vi "S8300E_WriteSN.vi"() -> ()   [LabVIEW 2011]
panel:
  out "log1":string
  out "Debug View":string
  out "UUT SN":string
  out "CMD-LIST":cluster{string, string, string, string}[](array[cluster])
  out "log msg":string
  out "VISA resource name out":refnum<visa-resource-name>
  out "BEGIN TIME":u32
  out "進行狀況":string
  # "2014-12-15"
  # "S8300E Program SN (接UART COM9)"
  # "Error Code:SN-SET"
  # "Set Serial Number to BIOS Flash"
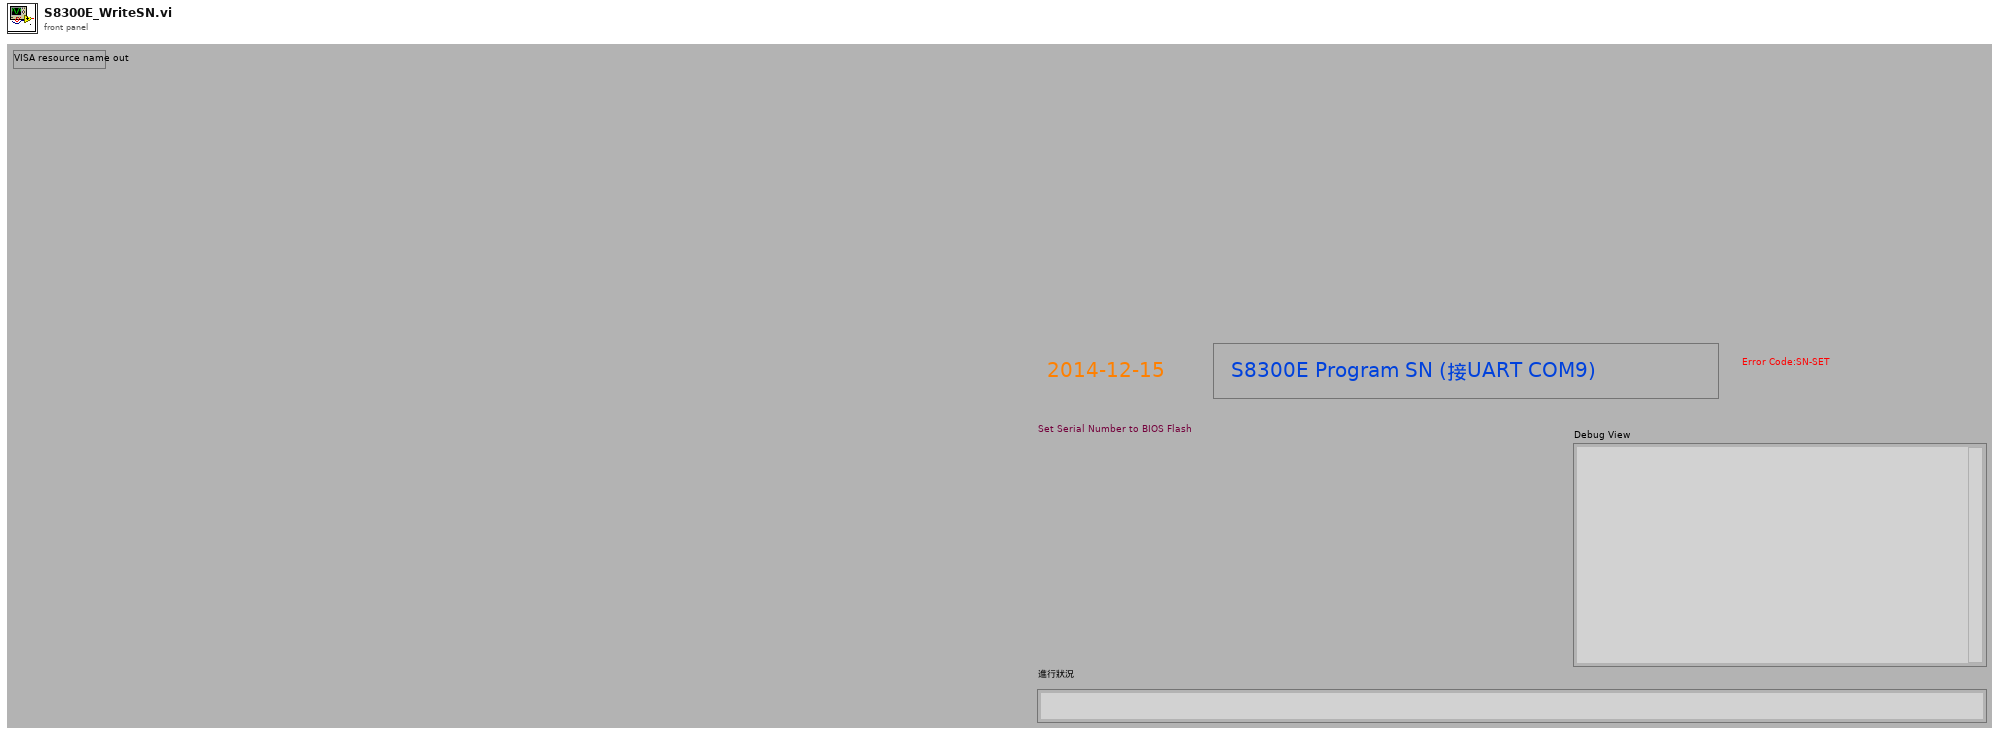
[diagram p1: front panel]
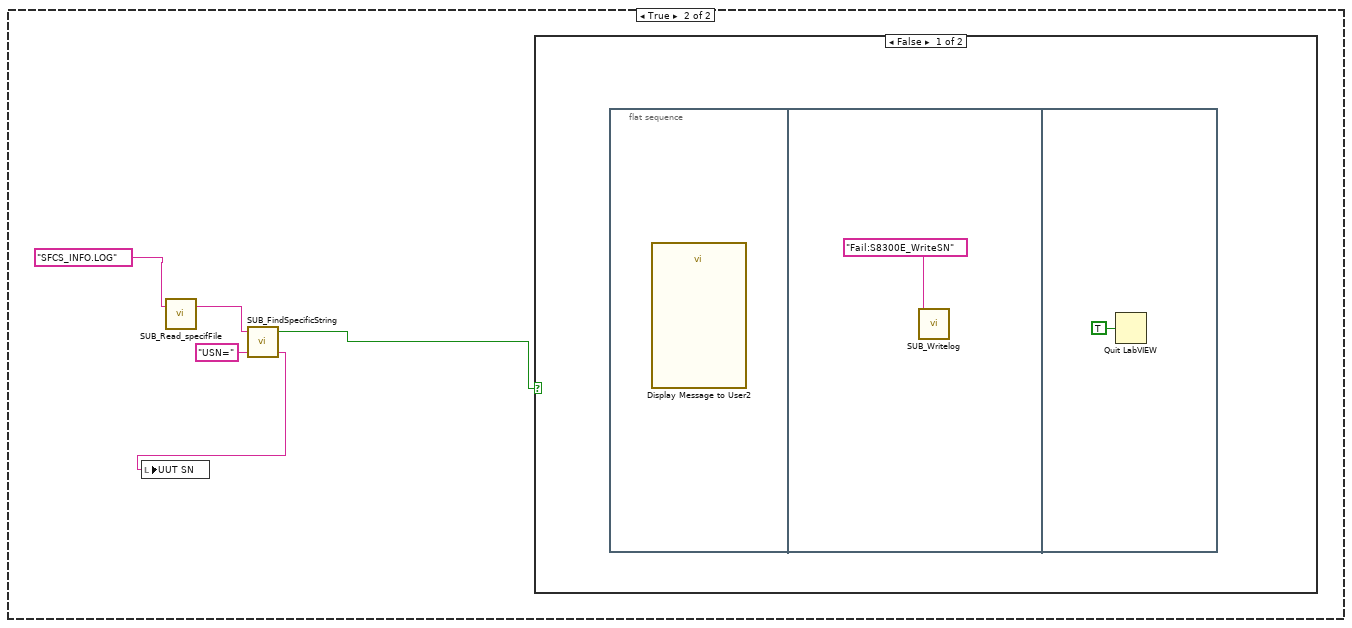
[diagram p3: hidden frame]
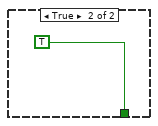
[diagram p7: hidden frame]
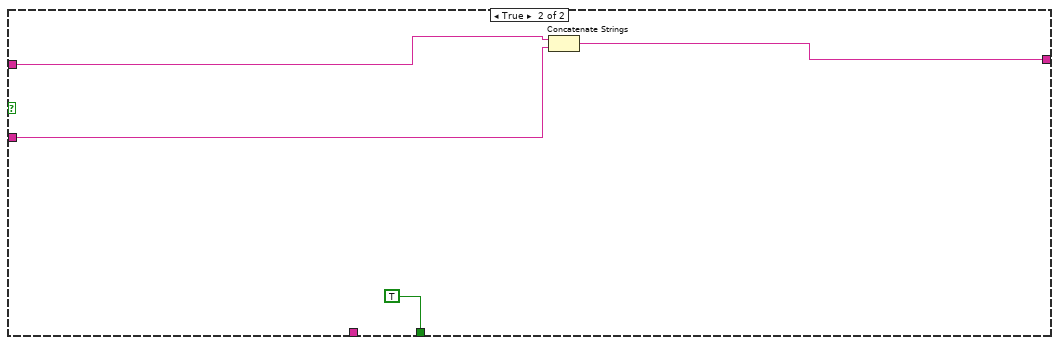
[diagram p9: hidden frame]
diagram:
  n1 = flat-sequence {
    frame #0 {
      n2 = Tick Count (ms)() -> (millisecond timer value=→"BEGIN TIME":u32)
    }
    frame #1 {
      w2 = ""
      n3 = property on="進行狀況" class="Str"("Blinking"=TRUE) -> ()  [unwired: 2 in, 2 out]
      "進行狀況" <- "進入測試準備中...." ("進行狀況")
      "UUT SN" <- w2
      "Debug View" <- w2
    }
    frame #2 {
      n4 = call "SUB_SearchFile_inFolder.vi"("Search Filename in Folder"="S8300E_sfcs_misc.txt") -> ("File Existing True/Flase"=w5:bool)  [unwired: 1 in]
      n5 = case shown="False" w5 {
        frame False {
          n6 = flat-sequence {
            frame #0 {
              n7 = call "Display Message to User"() -> ()  [unwired: 10 in, 2 out]
            }
            frame #1 {
              n8 = call "SUB_Writelog.vi"("Pass/Fail"="Fail:S8300E_WriteSN") -> ()  [unwired: 2 in]
            }
            frame #2 {
              n9 = Quit LabVIEW(quit? (T)=TRUE) -> ()
            }
          }
        }
        frame True {
        }
      }
    }
    frame #3 {
    }
    frame #4 {
      n10 = call "SUB_SearchFile_inFolder.vi"("Search Filename in Folder"="SFCS_INFO.LOG") -> ("File Existing True/Flase"=w9:bool)  [unwired: 1 in]
      n11 = case shown="False" w9 {
        frame False {
          n12 = flat-sequence {
            frame #0 {
              n13 = call "Display Message to User3"() -> ()  [unwired: 10 in, 2 out]
            }
            frame #1 {
              n14 = call "SUB_Writelog.vi"("Pass/Fail"="Fail:S8300E_WriteSN") -> ()  [unwired: 2 in]
            }
            frame #2 {
              n15 = Quit LabVIEW(quit? (T)=TRUE) -> ()
            }
          }
        }
        frame True {
          n16 = call "SUB_Read_specifFile.vi"("name or relative path"="SFCS_INFO.LOG" ("Search Filename in Folder")) -> ("text"=w16:string)  [unwired: 1 in, 1 out]
          n17 = call "SUB_FindSpecificString.vi"("Find this String"="USN=", "String data"=w16) -> ("before \"; \" string"=w14:string, "Found"=w13:bool)  [unwired: 2 in]
          n18 = local write "UUT SN"(w14) -> ()
          n19 = case shown="False" w13 {
            frame False {
              n20 = flat-sequence {
                frame #0 {
                  n21 = call "Display Message to User2"() -> ()  [unwired: 10 in, 2 out]
                }
                frame #1 {
                  n22 = call "SUB_Writelog.vi"("Pass/Fail"="Fail:S8300E_WriteSN") -> ()  [unwired: 2 in]
                }
                frame #2 {
                  n23 = Quit LabVIEW(quit? (T)=TRUE) -> ()
                }
              }
            }
            frame True {
            }
          }
        }
      }
    }
    frame #5 {
      n24 = local read "UUT SN"() -> (w23:string)
      n25 = Concatenate Strings("PASSED=", w23) -> (w22:string)
      n26 = Concatenate Strings("PASSED=", w23) -> (w25:string)
      n27 = Concatenate Strings("./ser.sh -w -f  ", w23, "\r") -> (w41:string)
      n28 = Concatenate Strings("./ser.sh -r -f  ", "\r") -> (w38:string)
      n29 = Concatenate Strings("./ser.sh -r -d ", "\r") -> (w35:string)
      n30 = Bundle(w41, "PASSED=", "Set Serial Number to BIOS Flash", "SN-SET") -> (w30:cluster{string, string, string, string})  [unwired: 1 in]
      n31 = Bundle(w38, w25, "Get Serial Number from BIOS Flash", "SN-BIOS") -> ()  [unwired: 1 in, 1 out]
      n32 = Bundle(w35, w22, "Get Serial Number from DMI table", "SN-DMI") -> ()  [unwired: 1 in, 1 out]
      n33 = Build Array(w30) -> (→"CMD-LIST":cluster{string, string, string, string}[])
    }
    frame #6 {
      n34 = call "SUB_COM1_CLOSE.vi"("VISA resource name"=refnum<visa-resource-name> "COM9") -> ()  [unwired: 3 in]
    }
    frame #7 {
      n35 = call "SUB_COM9_INIT.vi"("baud rate"=u32 115200) -> ("VISA resource name out"=w47:refnum<visa-resource-name>)  [unwired: 1 in, 1 out]
      "VISA resource name out" <- w47
      n36 = call "SUB_COM1Wrt.vi"("VISA resource name"=w47, "write buffer"="\r") -> ("duplicate VISA resource name"=w44:refnum<visa-resource-name>)  [unwired: 1 in, 1 out]
      n37 = call "SUB_ContinueCom1Read.vi"("Numeric"=1200, "duplicate VISA resource name 2"=w44) -> ()  [unwired: 1 in, 3 out]
    }
    frame #8 {
      n38 = case shown="True" TRUE {
        frame False {
        }
        frame True {
          n39 = while {
            stop <- w57 stop-if-true
            n40 = local read "VISA resource name out"() -> (w51:refnum<visa-resource-name>)
            n41 = call "SUB_COM1Wrt.vi"("VISA resource name"=w51, "write buffer"="\r") -> ("duplicate VISA resource name"=w56:refnum<visa-resource-name>)  [unwired: 1 in, 1 out]
            n42 = Tick Count (ms)() -> (millisecond timer value=w55:u32)
            n43 = call "SUB_READ_COM1_FindString_timeout.vi"("Find this String"="s8300e_func_test", "Timeout Seccond"=1.0, "Begin time"=w55, "duplicate VISA resource name 2"=w56) -> ("Output String"=w50:string, "Found String"=w52:bool)  [unwired: 1 in, 1 out]
            "log1" <- w50
            n44 = local write "Debug View"(w50) -> ()
            n45 = case shown="False" w52 {
              tunnel: [w60 TRUE] -> w57
              tunnel: w50 -> [w59 _]
              frame False {
                n46 = call "SUB_YESNO.vi"("Debug View"=w59, "Status"="UART無正確反應!需有S8300E字串") -> ("yes/no"=w63:enum32{"No Selection", "Yes", "No", "None"})  [unwired: 1 in]
                n47 = Equal?(x=w63, y=enum32{"No Selection", "Yes", "No", "None"}."No") -> (x = y?=w61:bool)
                n48 = case shown="True" w61 {
                  tunnel: [_ w65] -> w60
                  frame False {
                  }
                  frame True {
                    n49 = flat-sequence {
                      tunnel: [w69] -> w65
                      frame #0 {
                        n50 = call "SUB_Writelog.vi"("Pass/Fail"="Fail:S8300E_WriteSN") -> ()  [unwired: 2 in]
                      }
                      frame #1 {
                        n51 = call "SUB_SFCS_SendResult.vi"("ErrorCode"="UART", "PASS_Fail (1/0)"=i8 0) -> ()  [unwired: 1 out]
                      }
                      frame #2 {
                        w69 = TRUE ("quit? (T)")
                        n52 = Quit LabVIEW(quit? (T)=w69) -> ()
                      }
                    }
                  }
                }
              }
              frame True {
              }
            }
          }
        }
      }
    }
    frame #9 {
      n53 = local read "CMD-LIST"() -> (w71:cluster{string, string, string, string}[])
      n54 = Array Size(array=w71) -> (size(s)=w74:i32)
      n55 = for {
        N: w74 -> [_]
        shift-right: [w77] -> w72
        shift-left: "" -> [w76]
        i -> [w75]
        n56 = while {
          tunnel: w75 -> [w96]
          tunnel: [w90] -> w77
          tunnel: w76 -> [w89]
          stop <- w91 stop-if-true
          n57 = local read "VISA resource name out"() -> (w92:refnum<visa-resource-name>)
          n58 = local read "CMD-LIST"() -> (w88:cluster{string, string, string, string}[])
          n59 = Index Array(array=w88, index=w96) -> (element=w87:cluster{string, string, string, string})
          n60 = Unbundle(w87) -> (w86:string, w84:string, w85:string, w83:string)
          n61 = call "SUB_COM1Wrt.vi"("VISA resource name"=w92, "write buffer"=w86) -> ("duplicate VISA resource name"=w95:refnum<visa-resource-name>)  [unwired: 1 in, 1 out]
          n62 = Tick Count (ms)() -> (millisecond timer value=w94:u32)
          n63 = local read "UUT SN"() -> (w82:string)
          n64 = call "SUB_READ_COM1_FindString_timeout.vi"("Find this String"=w84, "Timeout Seccond"=3.0, "Begin time"=w94, "duplicate VISA resource name 2"=w95) -> ("Output String"=w78:string, "Found String"=w80:bool)  [unwired: 1 in, 1 out]
          n65 = call "SUB_FindSpecificString.vi"("Find this String"=w82, "String data"=w78) -> ("Found"=w79:bool)  [unwired: 2 in, 1 out]
          n66 = local write "進行狀況"(w85) -> ()
          n67 = local write "Debug View"(w78) -> ()
          n68 = And(x=w79, y=w80) -> (x .and. y?=w81:bool)
          n69 = case shown="False" w81 {
            tunnel: [_ TRUE] -> w91
            tunnel: w78 -> [w106 w112]
            tunnel: [w102 w114] -> w90
            tunnel: w89 -> [w102 w113]
            tunnel: w83 -> [w101 _]
            frame False {
              n70 = local read "進行狀況"() -> (w98:string)
              n71 = Concatenate Strings("失敗!" ("string"), "\r", w98) -> (w97:string)
              n72 = call "SUB_YESNO.vi"("Debug View"=w106, "Status"=w97) -> ("yes/no"=w105:enum32{"No Selection", "Yes", "No", "None"})  [unwired: 1 in]
              n73 = Equal?(x=w105, y=enum32{"No Selection", "Yes", "No", "None"}."No") -> (x = y?=w103:bool)
              n74 = case shown="True" w103 {
                tunnel: w101 -> [_ w107]
                frame False {
                }
                frame True {
                  n75 = flat-sequence {
                    tunnel: w107 -> [w108]
                    frame #0 {
                      n76 = call "SUB_SFCS_SendResult.vi"("ErrorCode"=w108, "PASS_Fail (1/0)"=i8 0) -> ()  [unwired: 1 out]
                    }
                    frame #1 {
                      n77 = call "SUB_Writelog.vi"("Pass/Fail"="Fail:S8300E_WriteSN") -> ()  [unwired: 2 in]
                    }
                    frame #2 {
                      n78 = Quit LabVIEW(quit? (T)=TRUE) -> ()
                    }
                  }
                }
              }
            }
            frame True {
              n79 = Concatenate Strings(w113, w112) -> (w114:string)
            }
          }
        }
      }
      "log msg" <- w72
    }
    frame #10 {
      w121 = "\n"
      n80 = local read "log1"() -> (w119:string)
      n81 = local read "log msg"() -> (w118:string)
      n82 = local read "BEGIN TIME"() -> (w125:u32)
      n83 = Tick Count (ms)() -> (millisecond timer value=w124:u32)
      n84 = call "SUB_COM1_CLOSE.vi"("VISA resource name"=refnum<visa-resource-name> "COM9") -> ()  [unwired: 3 in]
      n85 = Concatenate Strings(w119, w118) -> (w117:string)
      n86 = call "SUB_CAL_TESTTIME.vi"("Test Item name"="S8300E_WriteSN", "Stop tick time"=w124, "Start tick time"=w125) -> ("Test Time output"=w120:string)  [unwired: 2 in]
      n87 = Concatenate Strings("Pass:S8300E_WriteSN", w121, w117, w121, w120) -> (w123:string)
      n88 = call "SUB_Writelog.vi"("Pass/Fail"=w123) -> ()  [unwired: 2 in]
    }
    frame #11 {
      n89 = Request Deallocation(TRUE ("flag")) -> ()
    }
    frame #12 {
      n90 = Quit LabVIEW(quit? (T)=TRUE ("stop? (T)")) -> ()
    }
  }
